vi "Send Error Stream.vi"(8 "error in (no error)":errorcluster, 11 "Error Stream gRPCid":T1) -> (0 "error out":errorcluster)   [LabVIEW 2019]
uses:
  labview-grpc-query-server/VIs/MeasurementServer_gRPCid.ctl
  labview-grpc-query-server/VIs/MeasurementServer_ErrorOutData.ctl
  labview-grpc-query-server/VIs/labview-grpc-measurement-server.lvlib
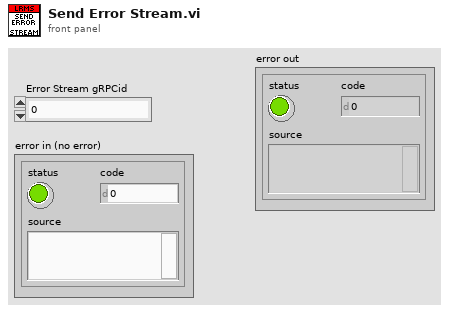
[diagram p1: front panel]
types:
  T1 = typedef "labview-grpc-measurement-server.lvlib/MeasurementServer_gRPCid.ctl" = u64
  T2 = typedef "labview-grpc-measurement-server.lvlib/MeasurementServer_ErrorOutData.ctl" = cluster{"ErrorCode":i32, "ErrorMessage":string}
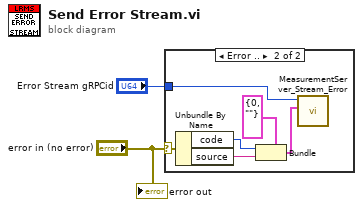
[diagram p0: block diagram]
diagram:
  n1 = case shown="Error .." "error in (no error)" {
    selector: "error in (no error)" -> [_ w8]
    tunnel: "Error Stream gRPCid" -> [_ w3]
    frame No Error {
    }
    frame Error {
      n2 = Unbundle By Name(w8) -> ("code"=w5:i32, "source"=w6:string)
      n3 = Bundle(cluster=T2 {"ErrorCode"=0, "ErrorMessage"=""} ("ErrorOutData"), "ErrorCode"=w5, "ErrorMessage"=w6) -> (w4:T2)
      n4 = call "MeasurementServer_Stream_Error.vi"("ErrorOutData"=w4, "gRPCid"=w3) -> ()  [unwired: 8 in, 2 out]
    }
  }
  "error out" <- "error in (no error)"
